vi "excitjob.vi"(0 "sample port":refnum<visa-resource-name>[](array[refnum]), 2 "sample sn":string[](array[string])) -> (7 "Array":bool[](array[boolean]), 8 "error":errorcluster[](array[cluster]))   [LabVIEW 2012]
uses:
  globalstatus.vi
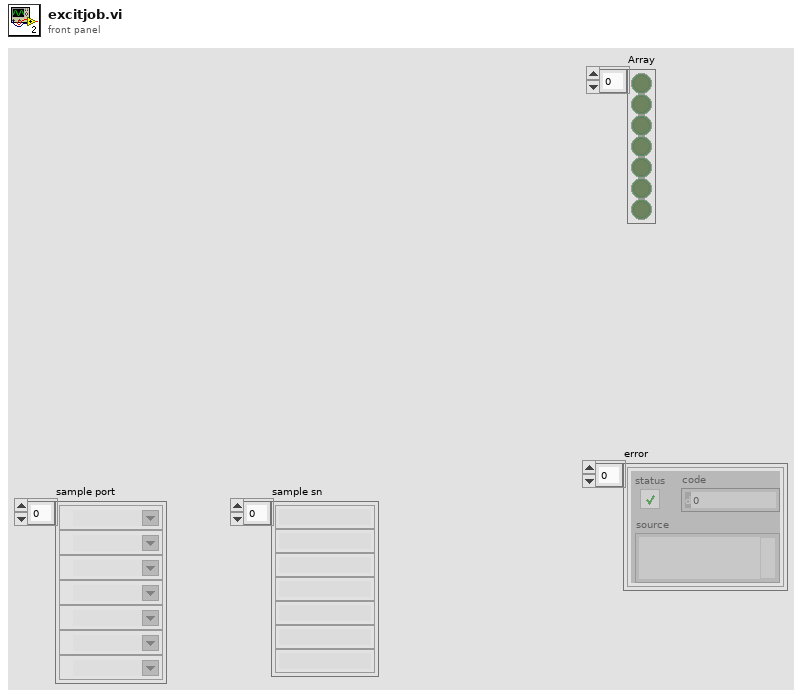
[diagram p1: front panel]
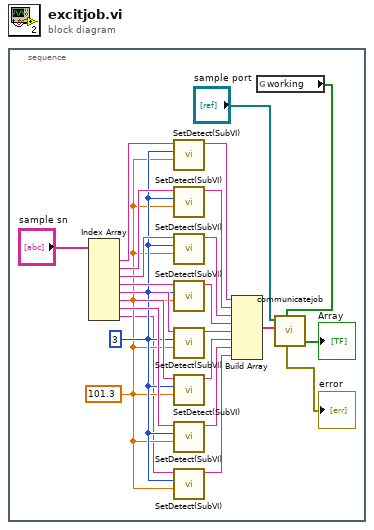
[diagram p0: block diagram]
diagram:
  n1 = stacked-sequence {
    frame #0 {
      w13 = 101.3
      w14 = 3
      n2 = Index Array(array="sample sn") -> (element #1=w23:string, element #2=w22:string, element #3=w21:string, element #4=w20:string, element #5=w19:string, element #6=w18:string, element #7=w15:string, element #8=w12:string)  [unwired: 8 in]
      n3 = call "SetDetect(SubVI).vi"("pressure"=w13, "led selected"=w14, "sn"=w23) -> ("output frame"=w9:string)  [unwired: 8 in]
      n4 = call "SetDetect(SubVI).vi"("pressure"=w13, "led selected"=w14, "sn"=w22) -> ("output frame"=w8:string)  [unwired: 8 in]
      n5 = call "SetDetect(SubVI).vi"("pressure"=w13, "led selected"=w14, "sn"=w21) -> ("output frame"=w7:string)  [unwired: 8 in]
      n6 = call "SetDetect(SubVI).vi"("pressure"=w13, "led selected"=w14, "sn"=w20) -> ("output frame"=w6:string)  [unwired: 8 in]
      n7 = call "SetDetect(SubVI).vi"("pressure"=w13, "led selected"=w14, "sn"=w19) -> ("output frame"=w2:string)  [unwired: 8 in]
      n8 = call "SetDetect(SubVI).vi"("pressure"=w13, "led selected"=w14, "sn"=w18) -> ("output frame"=w3:string)  [unwired: 8 in]
      n9 = call "SetDetect(SubVI).vi"("pressure"=w13, "led selected"=w14, "sn"=w15) -> ("output frame"=w4:string)  [unwired: 8 in]
      n10 = call "SetDetect(SubVI).vi"("pressure"=w13, "led selected"=w14, "sn"=w12) -> ("output frame"=w5:string)  [unwired: 8 in]
      n11 = Build Array(w9, w8, w7, w6, w2, w3, w4, w5) -> (w10:string[])
      n12 = global read "globalstatus.vi" "working"() -> (w1:bool[])
      n13 = call "communicatejob.vi"("sample port"="sample port", "condition"=w1, "send command"=w10) -> ("error"=→"error":errorcluster[], "receive result"=→"Array":bool[])  [unwired: 2 in, 2 out]
    }
  }
